vi "Read Buffer.vi"() -> ()   [LabVIEW 2015]
uses:
  <vilib>/FPGAPlugInAG/cRIO-9063/niLvFpga_Open_cRIO-9063.vi
  <vilib>/rvi/interface/common/dynamic/niFpgaDynamicAddResources.vi
  <vilib>/Utility/error.llb/Error Cluster From Error Code.vi
  <vilib>/rvi/errors/niLvFpgaAdjustHostInterfaceError.vi
  <vilib>/FPGAPlugInAG/Dynamic/niLvFpga_Run_Dynamic.vi
  <vilib>/FPGAPlugInAG/Dynamic/niLvFpga_Close_Dynamic.vi
  <vilib>/rvi/interface/nirviOpenFPGA/nirviOpenFPGA.xnode
  FPGA Bitfiles/VCU-VEHICLEMODEL_FPGATarget_CANBasic(FPGA)_WVt1gIpoBPw.lvbitx
  Basic (FPGA) CAN Engine .vi
  <vilib>/rvi/interface/nirviMethod/nirviMethod.xnode
  <vilib>/rvi/interface/nirviReadWriteControl/nirviReadWriteControl.xnode
  <vilib>/rvi/interface/nirviCloseFPGA/nirviCloseFPGA.xnode
  <vilib>/rvi/errors/niLvFpgaMergeErrorWithErrorCode.vi
  <vilib>/rvi/interface/Simulation/niFpgaSimulationCallBeginRW.vi
  NiFpgaLv.dll
  <vilib>/FPGAPlugInAG/Dynamic/niLvFpga_StartFifo_Dynamic.vi
  <vilib>/FPGAPlugInAG/Dynamic/niLvFpga_ReadFifo_Dynamic.vi
panel:
  out "Data":u32[](array[numeric])
  out "Overflow - Timed Out":bool
  in  "Stream":bool
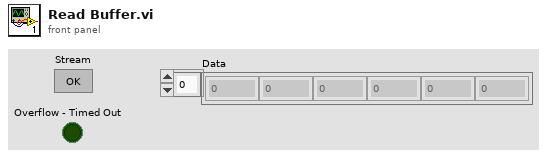
[diagram p1: front panel]
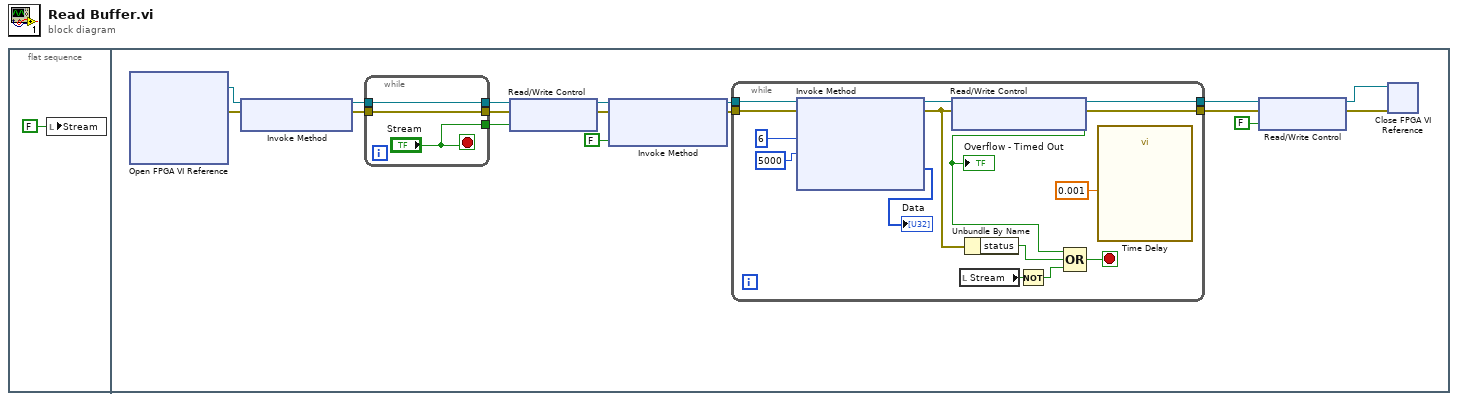
[diagram p0: block diagram]
diagram:
  n1 = flat-sequence {
    frame #0 {
      n2 = local write "Stream"(FALSE ("Stream")) -> ()
    }
    frame #1 {
      n3 = xnode "Open FPGA VI Reference"() -> ("FPGA VI Reference Out"=w14:refnum<k20>, "error out"=w15:errorcluster)  [unwired: 2 in]
      n4 = xnode "Invoke Method"("FPGA VI Reference In"=w14, "error in"=w15) -> ("FPGA VI Reference Out"=w13:refnum<k20>, "error out"=w12:errorcluster)
      n5 = while {
        tunnel: [w20] -> w18
        tunnel: [w21] -> w17
        tunnel: ["Stream"] -> w16
        tunnel: w13 -> [w21]
        tunnel: w12 -> [w20]
        stop <- "Stream" stop-if-true
      }
      n6 = xnode "Read/Write Control"("FPGA VI Reference In"=w17, "error in"=w18, "Log to buffer"=w16) -> ("FPGA VI Reference Out"=w11:refnum<k20>, "error out"=w9:errorcluster)
      n7 = xnode "Invoke Method"("FPGA VI Reference In"=w11, "error in"=w9, "Wait Until Done (F)"=FALSE) -> ("FPGA VI Reference Out"=w10:refnum<k20>, "error out"=w8:errorcluster)
      n8 = while {
        tunnel: w10 -> [w22]
        tunnel: w8 -> [w23]
        tunnel: [w25] -> w3
        tunnel: [w26] -> w6
        stop <- w32 stop-if-true
        n9 = xnode "Invoke Method"("FPGA VI Reference In"=w22, "error in"=w23, "Number of Elements"=u32 6, "Timeout (ms)"=5000) -> ("FPGA VI Reference Out"=w34:refnum<k20>, "error out"=w28:errorcluster, "Data"=→"Data":u32[])  [unwired: 1 out]
        n10 = xnode "Read/Write Control"("FPGA VI Reference In"=w34, "error in"=w28) -> ("FPGA VI Reference Out"=w26:refnum<k20>, "error out"=w25:errorcluster, "Overflow - Timed Out"=w24:bool)
        "Overflow - Timed Out" <- w24
        n11 = local read "Stream"() -> (w31:bool)
        n12 = Unbundle By Name(w28) -> ("status"=w33:bool)
        n13 = Not(x=w31) -> (.not. x?=w30:bool)
        n14 = Compound Arithmetic op=OR(w24, w33, w30) -> (w32:bool)
        n15 = call "Time Delay"("Delay Time (s)"=0.001) -> ()  [unwired: 10 in, 1 out]
      }
      n16 = xnode "Read/Write Control"("FPGA VI Reference In"=w6, "error in"=w3, "Log to buffer"=FALSE) -> ("FPGA VI Reference Out"=w5:refnum<k20>, "error out"=w4:errorcluster)
      n17 = xnode "Close FPGA VI Reference"("FPGA VI Reference In"=w5, "error in"=w4) -> ()  [unwired: 1 out]
    }
  }
